vi "solar_qtimer Process.vi"(10 "Queue":refnum<queue>, 11 "QTimer Name":string) -> ()   [LabVIEW 2018]
doc: "[DEPRECIATED] Each QTimer launches this process to handle periodic messages."
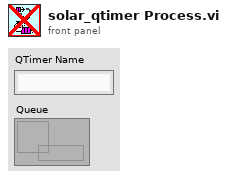
[diagram p1: front panel]
types:
  T1 = cluster{"msDelay":i32, "EnQ_Type":enum8{"Normal", "Priority", "IgnoreIfExists"}, "lastTime":u32, "Msg":cluster{"MSG":string, "DATA":variant}}
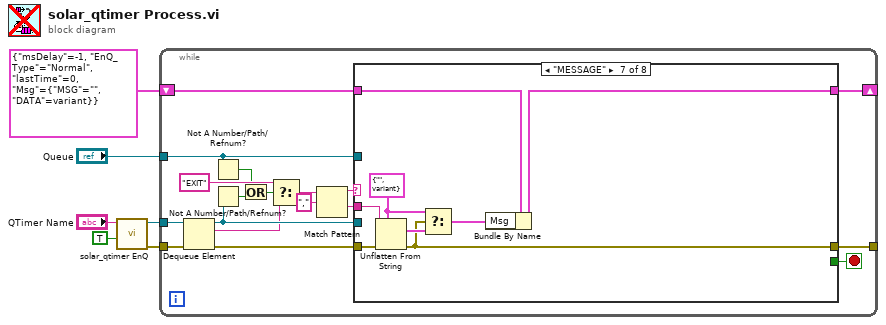
[diagram p0: block diagram]
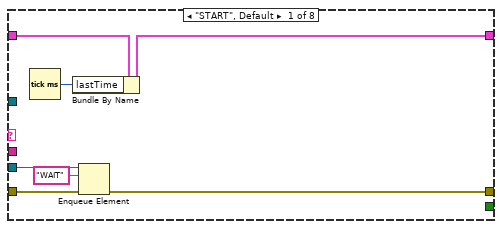
[diagram p2: hidden frame]
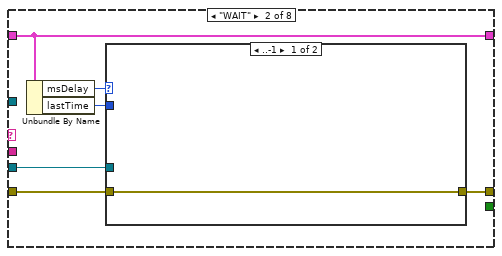
[diagram p3: hidden frame]
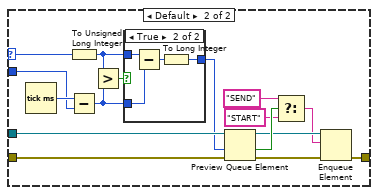
[diagram p4: hidden frame]
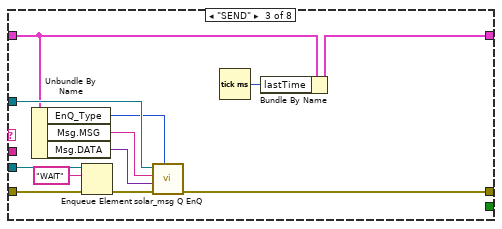
[diagram p6: hidden frame]
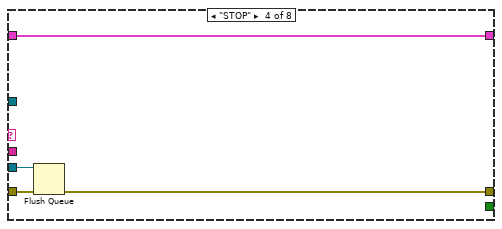
[diagram p7: hidden frame]
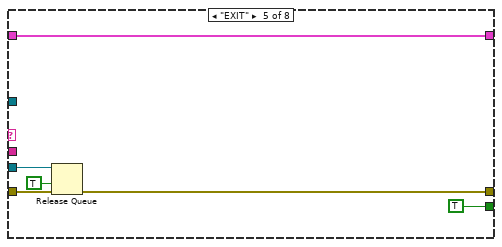
[diagram p8: hidden frame]
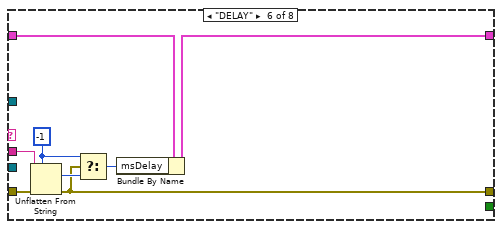
[diagram p9: hidden frame]
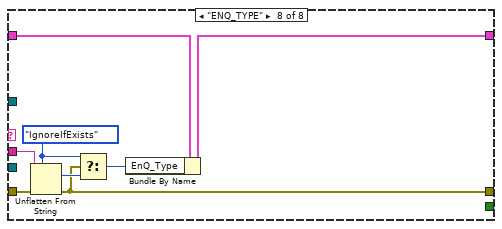
[diagram p10: hidden frame]
diagram:
  n1 = call "solar_qtimer EnQ.vi"("Create if not found? (F)"=TRUE, "QTimer Name"="QTimer Name") -> ("error out"=w5:errorcluster, "QTimer"=w6:refnum<queue>)  [unwired: 7 in, 1 out]
  n2 = while {
    tunnel: w6 -> [w24]
    tunnel: w5 -> [w23]
    tunnel: [w13] -> _
    shift-right: [w10] -> _
    shift-left: T1 {"msDelay"=-1, "EnQ_Type"=enum."Normal", "lastTime"=0, "Msg"={"MSG"="", "DATA"=variant}} ("QTimer Config") -> [w11]
    tunnel: "Queue" -> [w9]
    stop <- w12 stop-if-true
    n3 = Dequeue Element(queue=w24, error in (no error)=w23) -> (queue out=w18:refnum<queue>, element=w15:string, error out=w19:errorcluster)  [unwired: 1 in, 1 out]
    n4 = Not A Number/Path/Refnum?(number/path/refnum=w9) -> (NaN/Path/Refnum?=w7:bool)
    n5 = Not A Number/Path/Refnum?(number/path/refnum=w18) -> (NaN/Path/Refnum?=w17:bool)
    n6 = Or(x=w7, y=w17) -> (x .or. y?=w8:bool)
    n7 = Select(t="EXIT", s=w8, f=w15) -> (s? t:f=w14:string)
    n8 = Match Pattern(string=w14, regular expression=",") -> (before substring=w21:string, after substring=w20:string)  [unwired: 1 in, 2 out]
    n9 = case shown="\"MESSAGE\"" w21 {
      tunnel: w20 -> [_ _ _ _ _ w86 w94 w102]
      tunnel: w18 -> [w30 w34 w63 w73 w76 _ _ _]
      tunnel: w19 -> [w29 w33 w69 w72 w80 w87 w95 w103]
      tunnel: [w31 w32 w61 w71 w77 w83 w92 w100] -> w13
      tunnel: [_ _ _ _ TRUE _ _ _] -> w12
      tunnel: w11 -> [w26 w37 w68 w74 w78 w88 w96 w104]
      tunnel: [w28 w37 w66 w74 w78 w82 w91 w99] -> w10
      tunnel: w9 -> [_ _ w70 _ _ _ _ _]
      frame "START", Default {
        n10 = Tick Count (ms)() -> (millisecond timer value=w27:u32)
        n11 = Bundle By Name(cluster=w26, "lastTime"=w27) -> (w28:T1)
        n12 = Enqueue Element(queue=w30, element="WAIT", error in (no error)=w29) -> (error out=w31:errorcluster)  [unwired: 1 in, 2 out]
      }
      frame "WAIT" {
        n13 = Unbundle By Name(w37) -> ("msDelay"=w35:i32, "lastTime"=w36:u32)
        n14 = case shown="..-1" w35 {
          selector: w35 -> [_ w52]
          tunnel: w36 -> [_ w53]
          tunnel: w34 -> [_ w48]
          tunnel: w33 -> [w38 w47]
          tunnel: [w38 w40] -> w32
          frame ..-1 {
          }
          frame Default {
            n15 = Tick Count (ms)() -> (millisecond timer value=w54:u32)
            n16 = To Unsigned Long Integer(number=w52) -> (unsigned 32bit integer=w51:u32)
            n17 = Subtract(x=w54, y=w53) -> (x-y=w49:u32)
            n18 = Greater?(x=w51, y=w49) -> (0:w50:bool)
            n19 = case shown="True" w50 {
              tunnel: w51 -> [_ w58]
              tunnel: w49 -> [_ w57]
              tunnel: [_ w55] -> w46
              frame False {
              }
              frame True {
                n20 = Subtract(x=w58, y=w57) -> (x-y=w56:u32)
                n21 = To Long Integer(number=w56) -> (32bit integer=w55:i32)
              }
            }
            n22 = Preview Queue Element(queue=w48, timeout in ms (-1)=w46, error in (no error)=w47) -> (queue out=w42:refnum<queue>, timed out?=w45:bool, error out=w41:errorcluster)  [unwired: 1 out]
            n23 = Select(t="SEND", s=w45, f="START") -> (s? t:f=w39:string)
            n24 = Enqueue Element(queue=w42, element=w39, error in (no error)=w41) -> (error out=w40:errorcluster)  [unwired: 1 in, 2 out]
          }
        }
      }
      frame "SEND" {
        n25 = Unbundle By Name(w68) -> ("EnQ_Type"=w67:enum8{"Normal", "Priority", "IgnoreIfExists"}, "Msg.MSG"=w60:string, "Msg.DATA"=w59:variant)
        n26 = Enqueue Element(queue=w63, element="WAIT", error in (no error)=w69) -> (error out=w64:errorcluster)  [unwired: 1 in, 2 out]
        n27 = call "solar_msg Q EnQ.vi"("Priority (Normal)"=w67, "error in (no error)"=w64, "CMD_DATA (Last)"=w59, "CMD (Last)"=w60, "Queue in"=w70) -> ("error out"=w61:errorcluster)  [unwired: 4 in, 2 out]
        n28 = Tick Count (ms)() -> (millisecond timer value=w65:u32)
        n29 = Bundle By Name(cluster=w68, "lastTime"=w65) -> (w66:T1)
      }
      frame "STOP" {
        n30 = Flush Queue(queue=w73, error in (no error)=w72) -> (error out=w71:errorcluster)  [unwired: 2 out]
      }
      frame "EXIT" {
        n31 = Release Queue(queue=w76, force destroy? (F)=TRUE, error in (no error)=w80) -> (error out=w77:errorcluster)  [unwired: 2 out]
      }
      frame "DELAY" {
        w84 = -1
        n32 = Unflatten From String(type=w84, binary string=w86, error in (no error)=w87) -> (value=w85:i32, error out=w83:errorcluster)  [unwired: 2 in, 1 out]
        n33 = Select(t=w84, s=w83, f=w85) -> (s? t:f=w81:i32)
        n34 = Bundle By Name(cluster=w88, "msDelay"=w81) -> (w82:T1)
      }
      frame "MESSAGE" {
        w89 = cluster{"MSG":string, "DATA":variant} {"MSG"="", "DATA"=variant} ("Msg")
        n35 = Unflatten From String(type=w89, binary string=w94, error in (no error)=w95) -> (value=w93:cluster{"MSG":string, "DATA":variant}, error out=w92:errorcluster)  [unwired: 2 in, 1 out]
        n36 = Select(t=w89, s=w92, f=w93) -> (s? t:f=w90:cluster{"MSG":string, "DATA":variant})
        n37 = Bundle By Name(cluster=w96, "Msg"=w90) -> (w91:T1)
      }
      frame "ENQ_TYPE" {
        w97 = enum8{"Normal", "Priority", "IgnoreIfExists"}."IgnoreIfExists" ("EnQ_Type")
        n38 = Unflatten From String(type=w97, binary string=w102, error in (no error)=w103) -> (value=w101:enum8{"Normal", "Priority", "IgnoreIfExists"}, error out=w100:errorcluster)  [unwired: 2 in, 1 out]
        n39 = Select(t=w97, s=w100, f=w101) -> (s? t:f=w98:enum8{"Normal", "Priority", "IgnoreIfExists"})
        n40 = Bundle By Name(cluster=w104, "EnQ_Type"=w98) -> (w99:T1)
      }
    }
  }
